vi "AddTracepoint.vi"(8 "error in (no error)":errorcluster, 11 "tracepoint":string) -> (0 "error out":errorcluster)   [LabVIEW 2017, in "TraceLogger.lvlib"]
uses:
  <vilib>/addons/TraceLogger/TraceLogger.lvlib
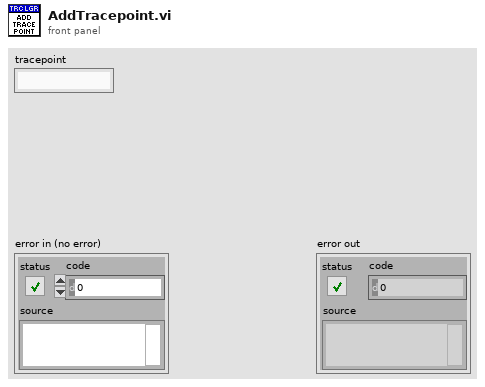
[diagram p1: front panel]
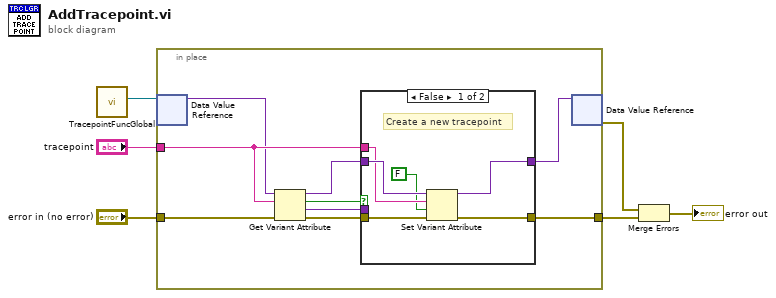
[diagram p0: block diagram]
diagram:
  n1 = call <vilib>:"TracepointFuncGlobal.vi"() -> ("tracepoints"=w5:refnum<data-value>)  [unwired: 11 in]
  n2 = in-place {
    in-place-border: "error in (no error)" -> [w15]
    in-place-border: [w13] -> w2
    in-place-border: "tracepoint" -> [w9]
    n3 = in-place-dvr #1(w5) -> (w8:variant)  [unwired: 1 out]
    n4 = Get Variant Attribute(Variant=w8, name=w9, error in=w15) -> (duplicate Variant=w10:variant, found=w11:bool, value=w12:variant, error out=w14:errorcluster)  [unwired: 1 in]
    n5 = case shown="False" w11 {
      tunnel: w14 -> [w21 w22]
      tunnel: [w20 w22] -> w13
      tunnel: w12 -> [_ _]
      tunnel: w10 -> [w19 w23]
      tunnel: w9 -> [w18 _]
      tunnel: [w16 w23] -> w7
      frame False {
        # "Create a new tracepoint"
        n6 = Set Variant Attribute(Variant=w19, name=w18, value=FALSE, error in=w21) -> (Variant out=w16:variant, error out=w20:errorcluster)  [unwired: 1 out]
      }
      frame True {
      }
    }
    n7 = in-place-dvr #1(w7) -> (w4:errorcluster)  [unwired: 1 out]
  }
  n8 = Merge Errors(w4, w2) -> (→"error out":errorcluster)
